vi "create tdms file.vi"(5 "task out":refnum<k21>, 7 "format":string="%<%y-%m-%d_%Hh%Mm%S>T.tdms", 9 "Application Directory":path) -> (0 "error out":errorcluster, 3 "tdms file out":refnum<k34>)   [LabVIEW 2010]
doc: "Creation d'un nouveau fichier TDMS selon le format donné en entrée."
uses:
  C:/Program Files/National Instruments/LabVIEW 2010/resource/objmgr/daqmx.rc
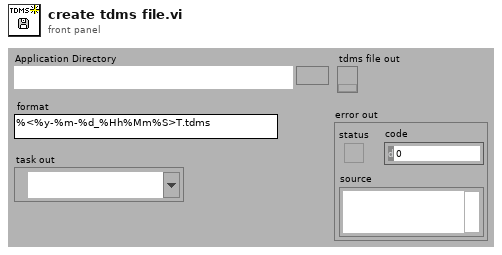
[diagram p1: front panel]
types:
  T1 = enum16{"open", "open or create", "create or replace", "create", "open (read-only)"}
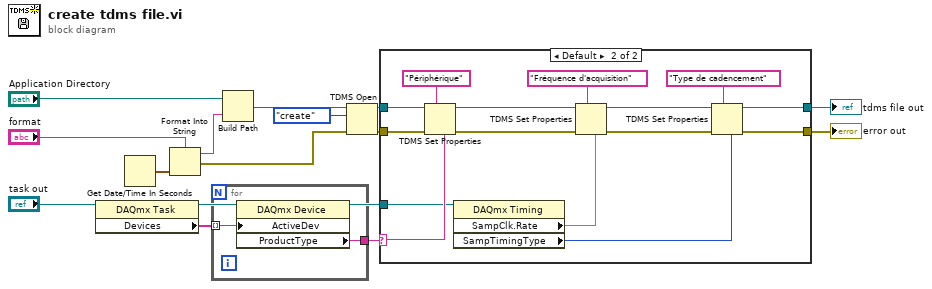
[diagram p0: block diagram]
diagram:
  n1 = property class="DAQmx Task"(reference="task out") -> (reference out=w3:refnum<k21>, "Devices"=w2:tag[])  [unwired: 1 in, 1 out]
  n2 = Get Date/Time In Seconds() -> (seconds since 1Jan1904=w14:timestamp)
  n3 = Format Into String(format string="format", w14) -> (resulting string=w13:string, error out=w9:errorcluster)  [unwired: 2 in]
  n4 = for {
    tunnel: w2 -> [w17] mode=indexing
    tunnel: [w16] -> w1
    n5 = property class="DAQmx Device"("ActiveDev"=w17) -> ("ProductType"=w16:string)  [unwired: 2 in, 2 out]
  }
  n6 = Build Path(base path="Application Directory", name or relative path=w13) -> (appended path=w11:path)
  n7 = TDMS Open(8:w9, 10:T1."create", 11:w11) -> (0:w6:errorcluster, 3:w8:refnum<k34>)  [unwired: 3 in]
  n8 = case shown="Default" w1 {
    selector: w1 -> [_ w32]
    tunnel: w8 -> [w19 w34]
    tunnel: [w19 w26] -> w7
    tunnel: w6 -> [w18 w33]
    tunnel: [w18 w23] -> w5
    tunnel: w3 -> [_ w22]
    frame "" {
    }
    frame Default {
      n9 = TDMS Set Properties(5:w32, 7:"Périphérique", 8:w33, 11:w34) -> (0:w25:errorcluster, 3:w28:refnum<k34>)  [unwired: 2 in, 2 out]
      n10 = property class="DAQmx Timing"(reference=w22) -> ("SampClk.Rate"=w21:dbl, "SampTimingType"=w20:i32)  [unwired: 1 in, 2 out]
      n11 = TDMS Set Properties(5:w21, 7:"Fréquence d'acquisition", 8:w25, 11:w28) -> (0:w24:errorcluster, 3:w27:refnum<k34>)  [unwired: 2 in, 2 out]
      n12 = TDMS Set Properties(5:w20, 7:"Type de cadencement", 8:w24, 11:w27) -> (0:w23:errorcluster, 3:w26:refnum<k34>)  [unwired: 2 in, 2 out]
    }
  }
  "error out" <- w5
  "tdms file out" <- w7
